vi "Update Status.vi"(8 "error in (no error)":errorcluster, 10 "Message":string, 11 "Status in":refnum<class "Status.lvclass">) -> (0 "error out":errorcluster, 3 "Status out":refnum<class "Status.lvclass">)   [LabVIEW 2020, in "neg-pkg.lvlib" / "Status.lvclass"]
uses:
  Status.lvclass
  Status Message Data.ctl
  Status.lvclass/Status.ctl
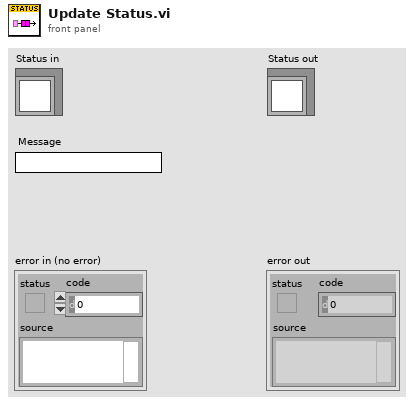
[diagram p1: front panel]
types:
  T1 = typedef "neg-pkg.lvlib/Status.lvclass/Status Message Data.ctl" = cluster{"Message":string}
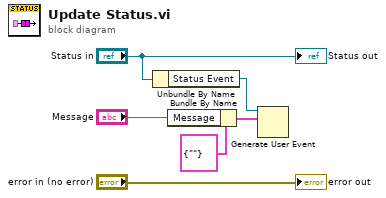
[diagram p0: block diagram]
diagram:
  n1 = Unbundle By Name("Status in") -> ("Status Event"=w4:refnum<user-event>)
  n2 = Bundle By Name(cluster=T1 {"Message"=""} ("Status Message Data"), "Message"="Message") -> (w1:T1)
  n3 = Generate User Event(user event=w4, event data cluster=w1) -> ()  [unwired: 2 in, 2 out]
  "error out" <- "error in (no error)"
  "Status out" <- "Status in"
